vi "Axis_Action Q.vi"(7 "Enum":enum16{"Initial", "Write", "Read"}(ring)=enum."Read", 8 "error in":errorcluster, 9 "Axis Index":i32, 10 "Axis ActFeedBackQ":refnum<queue>, 11 "Axis ActQ":refnum<queue>) -> (0 "error out":errorcluster, 2 "Axis ActFeedBackQ Out":refnum<queue>, 3 "Axis ActQ Out":refnum<queue>)   [LabVIEW 2019]
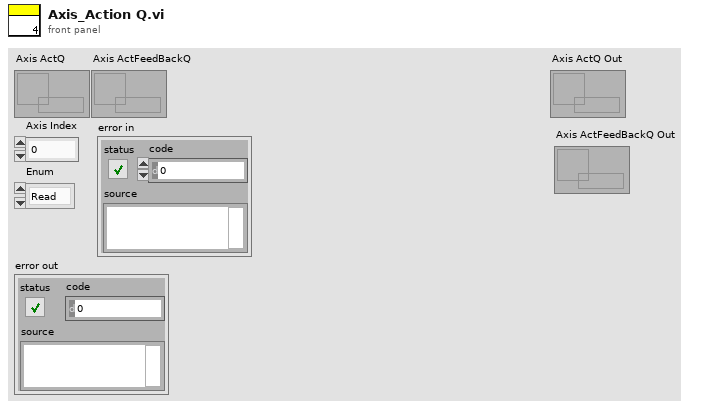
[diagram p1: front panel]
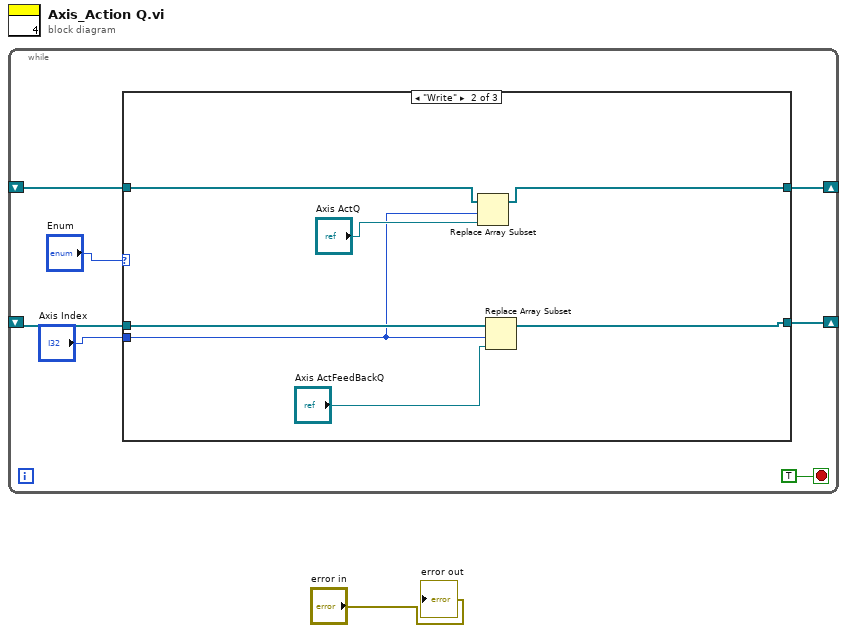
[diagram p0: block diagram]
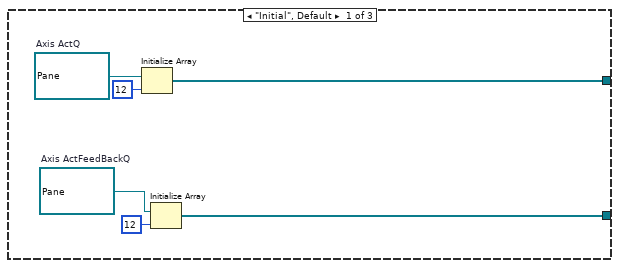
[diagram p2: hidden frame]
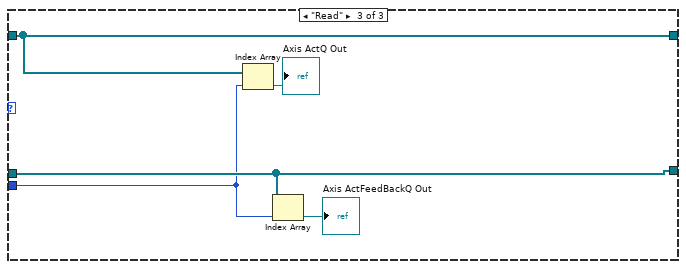
[diagram p3: hidden frame]
diagram:
  n1 = while {
    shift-right: [w6] -> _
    shift-left: _ -> [w4]
    shift-right: [w5] -> _
    shift-left: _ -> [w3]
    stop <- TRUE stop-if-true
    n2 = case shown="\"Write\"" "Enum" {
      tunnel: [w12 w20 w26] -> w6
      tunnel: [w9 w18 w25] -> w5
      tunnel: w4 -> [_ w21 w26]
      tunnel: w3 -> [_ w19 w25]
      tunnel: "Axis Index" -> [_ w15 w24]
      frame "Initial", Default {
        w10 = refnum<queue> refnum  # Axis ActFeedBackQ
        w14 = refnum<queue> refnum  # Axis ActQ
        n3 = Initialize Array(w14, 12 ("dimension size")) -> (w12:refnum<queue>[])
        n4 = Initialize Array(w10, 12 ("dimension size")) -> (w9:refnum<queue>[])
      }
      frame "Write" {
        n5 = Replace Array Subset(array=w21, new element="Axis ActQ", index=w15) -> (w20:refnum<queue>[])
        n6 = Replace Array Subset(array=w19, new element="Axis ActFeedBackQ", index=w15) -> (w18:refnum<queue>[])
      }
      frame "Read" {
        n7 = Index Array(array=w26, index=w24) -> (element=→"Axis ActQ Out":refnum<queue>)
        n8 = Index Array(array=w25, index=w24) -> (element=→"Axis ActFeedBackQ Out":refnum<queue>)
      }
    }
  }
  "error out" <- "error in"
